vi "Initial, set and read (20190220).vi"() -> ()   [LabVIEW 2017]
panel:
  in  "Go to Wavelength":dbl=500.0
  out "Mono status":bool=TRUE
  out "Current Wavelength":dbl=499.991 min=350.0 max=1100.0 step=1.0 format="%#.1f"
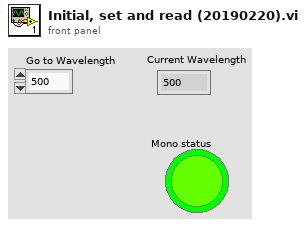
[diagram p1: front panel]
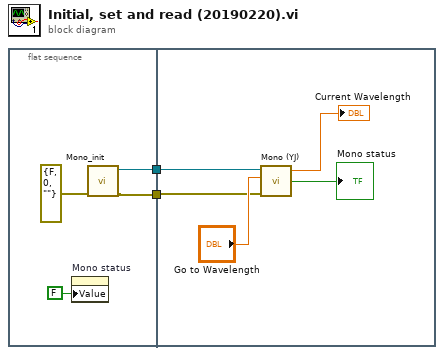
[diagram p0: block diagram]
diagram:
  n1 = flat-sequence {
    tunnel: [w5] -> w2
    tunnel: [w4] -> w1
    tunnel: w2 -> [w8]
    tunnel: w1 -> [w7]
    frame #0 {
      n2 = property on="Mono status" class="Bool (strict)"("Value"=FALSE ("Mono status")) -> ()  [unwired: 2 in, 2 out]
      n3 = call "Mono_init.vi"("error in (no error)"=errorcluster {"status"=FALSE, "code"=0, "source"=""}) -> ("error out"=w5:errorcluster, "CmdLib"=w4:refnum<k24>)  [unwired: 8 in, 1 out]
    }
    frame #1 {
      n4 = call "Mono (YJ).vi"("error in (no error)"=w8, "Go to Wavelength"="Go to Wavelength", "CmdLib In"=w7) -> ("State of Mono_SetWavelength"=→"Mono status":bool, "Current Wavelength"=→"Current Wavelength":dbl)  [unwired: 1 in, 1 out]
    }
  }
